vi "Extract Channels Preserve Value.vi"(6 "data type buffers in":T3, 7 "channel block":T1 {"buffer offset" format="%d bytes"}, 8 "error in (no error)":errorcluster, 9 "channels buffer index in":u64, 10 "channels buffer in":dbl[](array[numeric]), 11 "Buffer in":refnum<class "Buffer.lvclass">) -> (0 "error out":errorcluster, 1 "channels buffer index out":u64, 2 "channels buffer out":dbl[](array[numeric]), 3 "Buffer out":refnum<class "Buffer.lvclass">, 4 "data type buffers out":T3)   [LabVIEW 2017, in "DSF Core.lvlib" / "Buffer.lvclass"]
uses:
  Buffer.lvclass
  Typedefs/DSF Runtime Type Buffers.ctl
  Configuration/Public/Controls/DSF Engine Channel Configuration.ctl
  Configuration/Public/Controls/DSF Data Type.ctl
  Read 1D U64.vi
  Read 1D U32.vi
  Read 1D U16.vi
  Read 1D U8.vi
  Read 1D I64.vi
  Read 1D I32.vi
  Read 1D I16.vi
  Read 1D I8.vi
  Read 1D DBL.vi
  Read 1D SGL.vi
  Read 1D Bool.vi
  DSF Core.lvlib
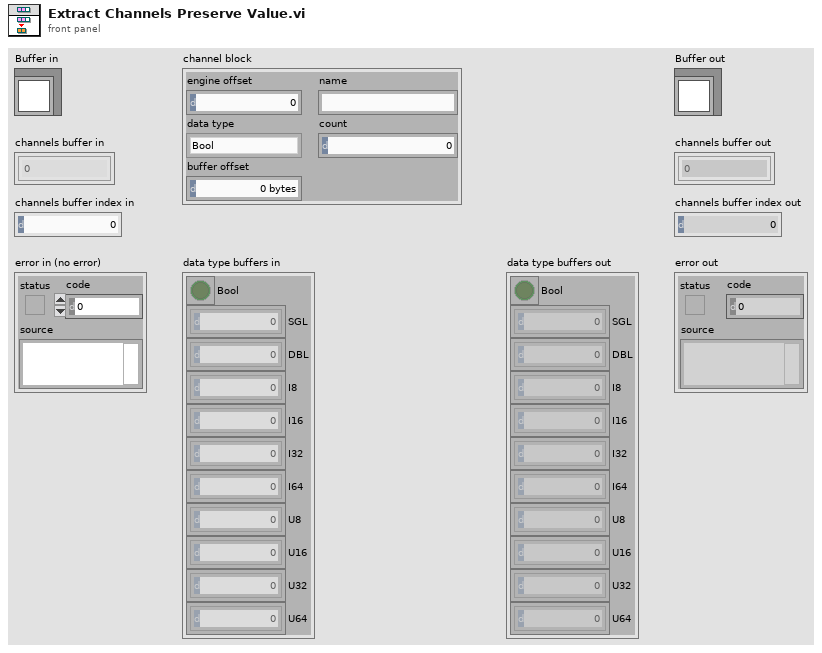
[diagram p1: front panel]
types:
  T1 = typedef "DSF Core.lvlib/DSF Engine Channel Configuration.ctl" = cluster{"engine offset":u64, "name":string, "data type":T2, "count":u64, "buffer offset":u64}
  T2 = typedef "DSF Core.lvlib/DSF Data Type.ctl" = enum8{"Bool", "SGL", "DBL", "I8", "I16", "I32", "I64", "U8", "U16", "U32", "U64"}
  T3 = typedef "DSF Core.lvlib/DSF Runtime Type Buffers.ctl" = cluster{"Bool":bool[], "SGL":sgl[], "DBL":dbl[], "I8":i8[], "I16":i16[], "I32":i32[], "I64":i64[], "U8":u8[], "U16":u16[], "U32":u32[], "U64":u64[]}
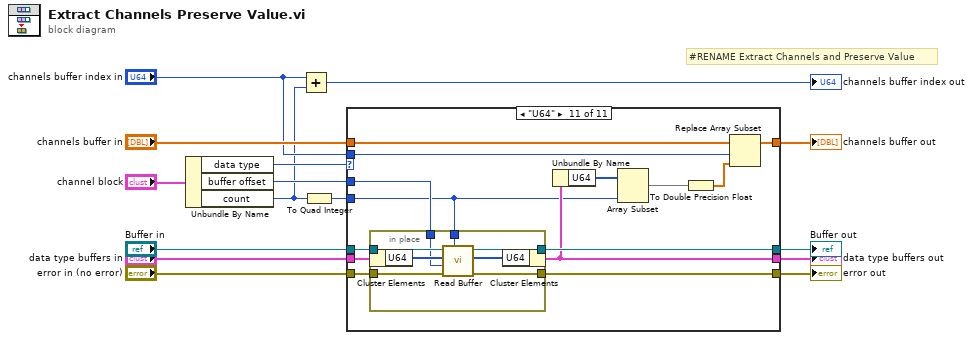
[diagram p0: block diagram]
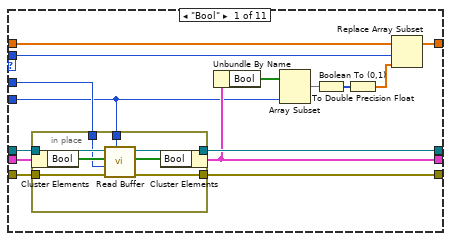
[diagram p2: hidden frame]
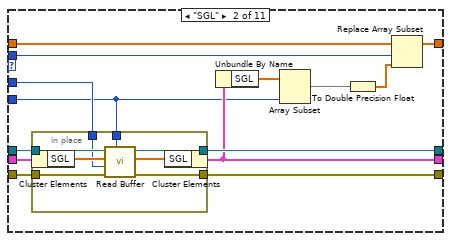
[diagram p3: hidden frame]
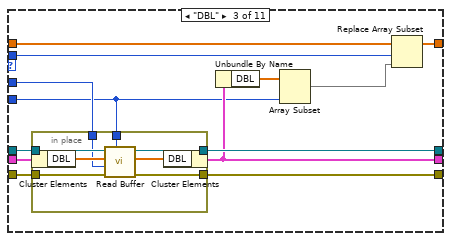
[diagram p4: hidden frame]
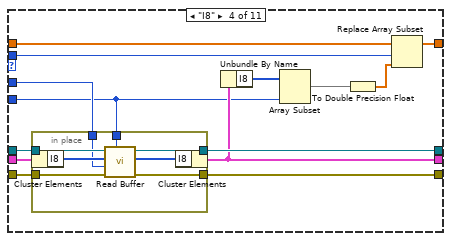
[diagram p5: hidden frame]
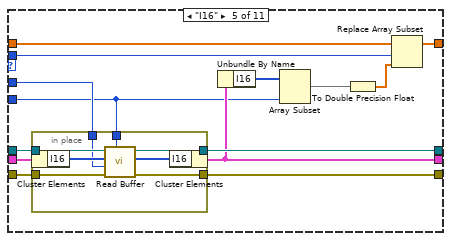
[diagram p6: hidden frame]
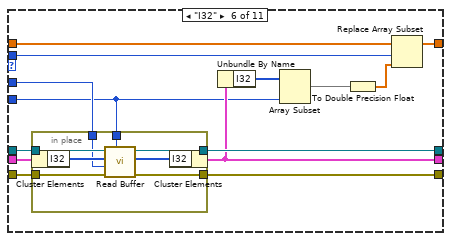
[diagram p7: hidden frame]
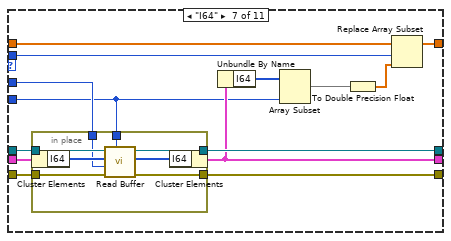
[diagram p8: hidden frame]
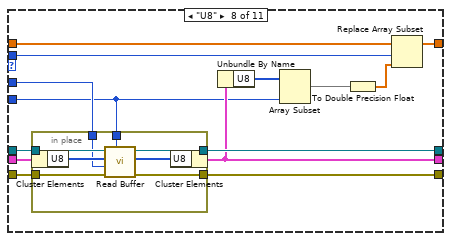
[diagram p9: hidden frame]
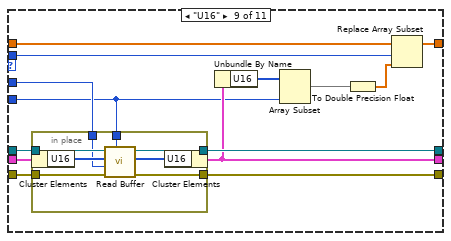
[diagram p10: hidden frame]
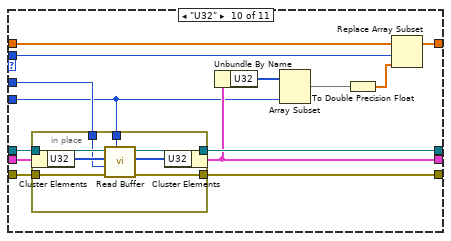
[diagram p11: hidden frame]
diagram:
  # "#RENAME Extract Channels and Preserve Value"
  n1 = Unbundle By Name("channel block") -> ("data type"=w13:T2, "buffer offset"=w3:u64, "count"=w1:u64)
  n2 = Add(x="channels buffer index in", y=w1) -> (x+y=→"channels buffer index out":u64)
  n3 = To Quad Integer(1:w1) -> (0:w8:i64)
  n4 = case shown="\"U64\"" w13 {
    tunnel: "Buffer in" -> [w30 w52 w73 w95 w117 w139 w161 w183 w205 w227 w249]
    tunnel: "error in (no error)" -> [w29 w51 w72 w94 w116 w138 w160 w182 w204 w226 w248]
    tunnel: [w28 w50 w71 w93 w115 w137 w159 w181 w203 w225 w247] -> w14
    tunnel: [w27 w49 w70 w92 w114 w136 w158 w180 w202 w224 w246] -> w11
    tunnel: "data type buffers in" -> [w26 w48 w69 w91 w113 w135 w157 w179 w201 w223 w245]
    tunnel: [w24 w46 w67 w89 w111 w133 w155 w177 w199 w221 w243] -> w9
    tunnel: w3 -> [w25 w47 w68 w90 w112 w134 w156 w178 w200 w222 w244]
    tunnel: w8 -> [w16 w40 w62 w83 w105 w127 w149 w171 w193 w215 w237]
    tunnel: "channels buffer in" -> [w20 w44 w65 w87 w109 w131 w153 w175 w197 w219 w241]
    tunnel: [w19 w43 w64 w86 w108 w130 w152 w174 w196 w218 w240] -> w6
    tunnel: "channels buffer index in" -> [w17 w41 w63 w84 w106 w128 w150 w172 w194 w216 w238]
    frame "Bool" {
      n5 = in-place {
        in-place-border: w30 -> [w38]
        in-place-border: w29 -> [w37]
        in-place-border: [w36] -> w28
        in-place-border: w25 -> [w32]
        in-place-border: [w35] -> w27
        in-place-border: w16 -> [w31]
        n6 = in-place-cluster #1(w26) -> ("Bool"=w34:bool[])
        n7 = call-poly "Read Buffer.vi"("count"=w31, "error in (no error)"=w37, "offset (0)"=w32, "buffer in"=w34, "Buffer in"=w38) -> ("error out"=w36:errorcluster, "buffer out"=w33:bool[], "Buffer out"=w35:refnum<class "Buffer.lvclass">)  [unwired: 3 in, 1 out]
        n8 = in-place-cluster #1("Bool"=w33) -> (w24:T3)
      }
      n9 = Unbundle By Name(w24) -> ("Bool"=w23:bool[])
      n10 = Array Subset(array=w23, length=w16) -> (w22:bool[])  [unwired: 1 in]
      n11 = Boolean To (0,1)(Boolean=w22) -> (0, 1=w21:i16[])
      n12 = To Double Precision Float(number=w21) -> (double precision float=w18:dbl[])
      n13 = Replace Array Subset(array=w20, new element=w18, index=w17) -> (w19:dbl[])
    }
    frame "SGL" {
      n14 = in-place {
        in-place-border: w52 -> [w60]
        in-place-border: w51 -> [w59]
        in-place-border: [w58] -> w50
        in-place-border: w47 -> [w54]
        in-place-border: [w57] -> w49
        in-place-border: w40 -> [w53]
        n15 = in-place-cluster #2(w48) -> ("SGL"=w56:sgl[])
        n16 = call-poly "Read Buffer.vi"("count"=w53, "error in (no error)"=w59, "offset (0)"=w54, "buffer in"=w56, "Buffer in"=w60) -> ("error out"=w58:errorcluster, "buffer out"=w55:sgl[], "Buffer out"=w57:refnum<class "Buffer.lvclass">)  [unwired: 3 in, 1 out]
        n17 = in-place-cluster #2("SGL"=w55) -> (w46:T3)
      }
      n18 = Unbundle By Name(w46) -> ("SGL"=w45:sgl[])
      n19 = Array Subset(array=w45, length=w40) -> (w39:sgl[])  [unwired: 1 in]
      n20 = To Double Precision Float(number=w39) -> (double precision float=w42:dbl[])
      n21 = Replace Array Subset(array=w44, new element=w42, index=w41) -> (w43:dbl[])
    }
    frame "DBL" {
      n22 = in-place {
        in-place-border: w73 -> [w81]
        in-place-border: w72 -> [w80]
        in-place-border: [w79] -> w71
        in-place-border: w68 -> [w75]
        in-place-border: [w78] -> w70
        in-place-border: w62 -> [w74]
        n23 = in-place-cluster #3(w69) -> ("DBL"=w77:dbl[])
        n24 = call-poly "Read Buffer.vi"("count"=w74, "error in (no error)"=w80, "offset (0)"=w75, "buffer in"=w77, "Buffer in"=w81) -> ("error out"=w79:errorcluster, "buffer out"=w76:dbl[], "Buffer out"=w78:refnum<class "Buffer.lvclass">)  [unwired: 3 in, 1 out]
        n25 = in-place-cluster #3("DBL"=w76) -> (w67:T3)
      }
      n26 = Unbundle By Name(w67) -> ("DBL"=w66:dbl[])
      n27 = Array Subset(array=w66, length=w62) -> (w61:dbl[])  [unwired: 1 in]
      n28 = Replace Array Subset(array=w65, new element=w61, index=w63) -> (w64:dbl[])
    }
    frame "I8" {
      n29 = in-place {
        in-place-border: w95 -> [w103]
        in-place-border: w94 -> [w102]
        in-place-border: [w101] -> w93
        in-place-border: w90 -> [w97]
        in-place-border: [w100] -> w92
        in-place-border: w83 -> [w96]
        n30 = in-place-cluster #4(w91) -> ("I8"=w99:i8[])
        n31 = call-poly "Read Buffer.vi"("count"=w96, "error in (no error)"=w102, "offset (0)"=w97, "buffer in"=w99, "Buffer in"=w103) -> ("error out"=w101:errorcluster, "buffer out"=w98:i8[], "Buffer out"=w100:refnum<class "Buffer.lvclass">)  [unwired: 3 in, 1 out]
        n32 = in-place-cluster #4("I8"=w98) -> (w89:T3)
      }
      n33 = Unbundle By Name(w89) -> ("I8"=w88:i8[])
      n34 = Array Subset(array=w88, length=w83) -> (w82:i8[])  [unwired: 1 in]
      n35 = To Double Precision Float(number=w82) -> (double precision float=w85:dbl[])
      n36 = Replace Array Subset(array=w87, new element=w85, index=w84) -> (w86:dbl[])
    }
    frame "I16" {
      n37 = in-place {
        in-place-border: w117 -> [w125]
        in-place-border: w116 -> [w124]
        in-place-border: [w123] -> w115
        in-place-border: w112 -> [w119]
        in-place-border: [w122] -> w114
        in-place-border: w105 -> [w118]
        n38 = in-place-cluster #5(w113) -> ("I16"=w121:i16[])
        n39 = call-poly "Read Buffer.vi"("count"=w118, "error in (no error)"=w124, "offset (0)"=w119, "buffer in"=w121, "Buffer in"=w125) -> ("error out"=w123:errorcluster, "buffer out"=w120:i16[], "Buffer out"=w122:refnum<class "Buffer.lvclass">)  [unwired: 3 in, 1 out]
        n40 = in-place-cluster #5("I16"=w120) -> (w111:T3)
      }
      n41 = Unbundle By Name(w111) -> ("I16"=w110:i16[])
      n42 = Array Subset(array=w110, length=w105) -> (w104:i16[])  [unwired: 1 in]
      n43 = To Double Precision Float(number=w104) -> (double precision float=w107:dbl[])
      n44 = Replace Array Subset(array=w109, new element=w107, index=w106) -> (w108:dbl[])
    }
    frame "I32" {
      n45 = in-place {
        in-place-border: w139 -> [w147]
        in-place-border: w138 -> [w146]
        in-place-border: [w145] -> w137
        in-place-border: w134 -> [w141]
        in-place-border: [w144] -> w136
        in-place-border: w127 -> [w140]
        n46 = in-place-cluster #6(w135) -> ("I32"=w143:i32[])
        n47 = call-poly "Read Buffer.vi"("count"=w140, "error in (no error)"=w146, "offset (0)"=w141, "buffer in"=w143, "Buffer in"=w147) -> ("error out"=w145:errorcluster, "buffer out"=w142:i32[], "Buffer out"=w144:refnum<class "Buffer.lvclass">)  [unwired: 3 in, 1 out]
        n48 = in-place-cluster #6("I32"=w142) -> (w133:T3)
      }
      n49 = Unbundle By Name(w133) -> ("I32"=w132:i32[])
      n50 = Array Subset(array=w132, length=w127) -> (w126:i32[])  [unwired: 1 in]
      n51 = To Double Precision Float(number=w126) -> (double precision float=w129:dbl[])
      n52 = Replace Array Subset(array=w131, new element=w129, index=w128) -> (w130:dbl[])
    }
    frame "I64" {
      n53 = in-place {
        in-place-border: w161 -> [w169]
        in-place-border: w160 -> [w168]
        in-place-border: [w167] -> w159
        in-place-border: w156 -> [w163]
        in-place-border: [w166] -> w158
        in-place-border: w149 -> [w162]
        n54 = in-place-cluster #7(w157) -> ("I64"=w165:i64[])
        n55 = call-poly "Read Buffer.vi"("count"=w162, "error in (no error)"=w168, "offset (0)"=w163, "buffer in"=w165, "Buffer in"=w169) -> ("error out"=w167:errorcluster, "buffer out"=w164:i64[], "Buffer out"=w166:refnum<class "Buffer.lvclass">)  [unwired: 3 in, 1 out]
        n56 = in-place-cluster #7("I64"=w164) -> (w155:T3)
      }
      n57 = Unbundle By Name(w155) -> ("I64"=w154:i64[])
      n58 = Array Subset(array=w154, length=w149) -> (w148:i64[])  [unwired: 1 in]
      n59 = To Double Precision Float(number=w148) -> (double precision float=w151:dbl[])
      n60 = Replace Array Subset(array=w153, new element=w151, index=w150) -> (w152:dbl[])
    }
    frame "U8" {
      n61 = in-place {
        in-place-border: w183 -> [w191]
        in-place-border: w182 -> [w190]
        in-place-border: [w189] -> w181
        in-place-border: w178 -> [w185]
        in-place-border: [w188] -> w180
        in-place-border: w171 -> [w184]
        n62 = in-place-cluster #8(w179) -> ("U8"=w187:u8[])
        n63 = call-poly "Read Buffer.vi"("count"=w184, "error in (no error)"=w190, "offset (0)"=w185, "buffer in"=w187, "Buffer in"=w191) -> ("error out"=w189:errorcluster, "buffer out"=w186:u8[], "Buffer out"=w188:refnum<class "Buffer.lvclass">)  [unwired: 3 in, 1 out]
        n64 = in-place-cluster #8("U8"=w186) -> (w177:T3)
      }
      n65 = Unbundle By Name(w177) -> ("U8"=w176:u8[])
      n66 = Array Subset(array=w176, length=w171) -> (w170:u8[])  [unwired: 1 in]
      n67 = To Double Precision Float(number=w170) -> (double precision float=w173:dbl[])
      n68 = Replace Array Subset(array=w175, new element=w173, index=w172) -> (w174:dbl[])
    }
    frame "U16" {
      n69 = in-place {
        in-place-border: w205 -> [w213]
        in-place-border: w204 -> [w212]
        in-place-border: [w211] -> w203
        in-place-border: w200 -> [w207]
        in-place-border: [w210] -> w202
        in-place-border: w193 -> [w206]
        n70 = in-place-cluster #9(w201) -> ("U16"=w209:u16[])
        n71 = call-poly "Read Buffer.vi"("count"=w206, "error in (no error)"=w212, "offset (0)"=w207, "buffer in"=w209, "Buffer in"=w213) -> ("error out"=w211:errorcluster, "buffer out"=w208:u16[], "Buffer out"=w210:refnum<class "Buffer.lvclass">)  [unwired: 3 in, 1 out]
        n72 = in-place-cluster #9("U16"=w208) -> (w199:T3)
      }
      n73 = Unbundle By Name(w199) -> ("U16"=w198:u16[])
      n74 = Array Subset(array=w198, length=w193) -> (w192:u16[])  [unwired: 1 in]
      n75 = To Double Precision Float(number=w192) -> (double precision float=w195:dbl[])
      n76 = Replace Array Subset(array=w197, new element=w195, index=w194) -> (w196:dbl[])
    }
    frame "U32" {
      n77 = in-place {
        in-place-border: w227 -> [w235]
        in-place-border: w226 -> [w234]
        in-place-border: [w233] -> w225
        in-place-border: w222 -> [w229]
        in-place-border: [w232] -> w224
        in-place-border: w215 -> [w228]
        n78 = in-place-cluster #10(w223) -> ("U32"=w231:u32[])
        n79 = call-poly "Read Buffer.vi"("count"=w228, "error in (no error)"=w234, "offset (0)"=w229, "buffer in"=w231, "Buffer in"=w235) -> ("error out"=w233:errorcluster, "buffer out"=w230:u32[], "Buffer out"=w232:refnum<class "Buffer.lvclass">)  [unwired: 3 in, 1 out]
        n80 = in-place-cluster #10("U32"=w230) -> (w221:T3)
      }
      n81 = Unbundle By Name(w221) -> ("U32"=w220:u32[])
      n82 = Array Subset(array=w220, length=w215) -> (w214:u32[])  [unwired: 1 in]
      n83 = To Double Precision Float(number=w214) -> (double precision float=w217:dbl[])
      n84 = Replace Array Subset(array=w219, new element=w217, index=w216) -> (w218:dbl[])
    }
    frame "U64" {
      n85 = in-place {
        in-place-border: w249 -> [w257]
        in-place-border: w248 -> [w256]
        in-place-border: [w255] -> w247
        in-place-border: w244 -> [w251]
        in-place-border: [w254] -> w246
        in-place-border: w237 -> [w250]
        n86 = in-place-cluster #11(w245) -> ("U64"=w253:u64[])
        n87 = call-poly "Read Buffer.vi"("count"=w250, "error in (no error)"=w256, "offset (0)"=w251, "buffer in"=w253, "Buffer in"=w257) -> ("error out"=w255:errorcluster, "buffer out"=w252:u64[], "Buffer out"=w254:refnum<class "Buffer.lvclass">)  [unwired: 3 in, 1 out]
        n88 = in-place-cluster #11("U64"=w252) -> (w243:T3)
      }
      n89 = Unbundle By Name(w243) -> ("U64"=w242:u64[])
      n90 = Array Subset(array=w242, length=w237) -> (w236:u64[])  [unwired: 1 in]
      n91 = To Double Precision Float(number=w236) -> (double precision float=w239:dbl[])
      n92 = Replace Array Subset(array=w241, new element=w239, index=w238) -> (w240:dbl[])
    }
  }
  "error out" <- w14
  "Buffer out" <- w11
  "channels buffer out" <- w6
  "data type buffers out" <- w9
